vi "HandlingLargeDataset.vi"() -> ()   [LabVIEW 2019]
uses:
  <vilib>/addons/database/Connection.llb/DB Tools Open Connec (String).vi
  <vilib>/addons/database/Connection.llb/Conn Execute.vi
  <vilib>/addons/database/Recordset.llb/Rec Fetch Recordset Data (R).vi
  <vilib>/addons/database/_DB Variant To Data/Database Variant To Data.xnode
  <vilib>/addons/database/NI_Database_API.lvlib
panel:
  out "graph refreshed or not":bool
  out "x+y":timestamp
  out "element":timestamp
  out "max Date 1Hour":timestamp
  out "max Date 1 Month":timestamp
  out "max Date 1 week":timestamp
  out "max Date 30 minutes":timestamp
  out "max Date 1 Minute":timestamp
  out "max date 1Day":timestamp
  out "Horizontal":i32
  in  "To Date":timestamp
  in  "from Date":timestamp
  in  "Stop Button":bool
  in  "DateTime Array for One Month":timestamp[](array[timestamp])
  in  "Length Array for One Month":dbl[](array[numeric])
  out "concatenated string 8":string
  in  "DateTime Array for one week":timestamp[](array[timestamp])
  in  "Length Array for One week":dbl[](array[numeric])
  out "concatenated string 7":string
  in  "DateTime Array for 1 Day":timestamp[](array[timestamp])
  in  "Length Array for 1 Day":dbl[](array[numeric])
  out "concatenated string 6":string
  in  "DateTime Array for 1 Hour":timestamp[](array[timestamp])
  in  "Length Array for 1 Hour":dbl[](array[numeric])
  out "concatenated string 5":string
  out "concatenated string 2":string
  out "concatenated string":string
  out "Currently active btn":string
  in  "DateTime Array for 30 mins":timestamp[](array[timestamp])
  in  "Length Array for 30 mins":dbl[](array[numeric])
  out "record set data for 30 minutes":variant[][](array[variant])
  out "Month  3":string
  out "Day  3":string
  out "year  3":string
  out "Month  2":string
  out "Day  2":string
  out "year  2":string
  out "concatenated string 4":string
  out "NewVal":bool
  out "output cluster":T1
  out "DateTime Array  2":timestamp[](array[timestamp])
  in  "Length Array":dbl[](array[numeric])
  in  "DateTime Array":timestamp[](array[timestamp])
  out "size(s)":i32[](array[numeric])
  out "Month  2":string
  out "Day  2":string
  out "year  2":string
  out "Month":string
  out "Day":string
  out "year":string
  out "concatenated string 3":string
  in  "1Hour":bool
  in  "30Minute":bool
  in  "OneMinute":bool caption="One Minute"
  out "ZooM":T2(graph)
  in  "One Month":bool
  in  "One Week":bool
  in  "One Day":bool
  out "Tota records":variant[][](array[variant])
  out "Program start time":timestamp
  # "Welcome to History Section  for Data Analysis"
  # "One Week"
types:
  T1 = cluster{"DateTime Array ":timestamp[], "Length Array ":dbl[]}
  T2 = cluster{"DateTime from Db ":timestamp[], "start from Db ":dbl[]}
  T3 = typedef "LVPoint32TypeDef.ctl" = cluster{"Horizontal":i32, "Vertical":i32}
  T4 = typedef "NI_Database_API.lvlib/Conn ObjectReference.ctl" = refnum<k1>
  T5 = typedef "NI_Database_API.lvlib/Rec ObjectReference.ctl" = refnum<k1>
  T6 = cluster{"DateTime Array for 30 mins ":timestamp[], "Length Array for 30 mins ":dbl[]}
  T7 = cluster{"DateTime Array for one week ":timestamp[], "Length Array for One week":dbl[]}
  T8 = cluster{"DateTime Array for One Month ":timestamp[], "Length Array for One Month ":dbl[]}
  T9 = cluster{"DateTime Array for 1 Hour ":timestamp[], "Length Array for 1 Hour ":dbl[]}
  T10 = cluster{"DateTime Array for 1 Day ":timestamp[], "Length Array for 1 Day ":dbl[]}
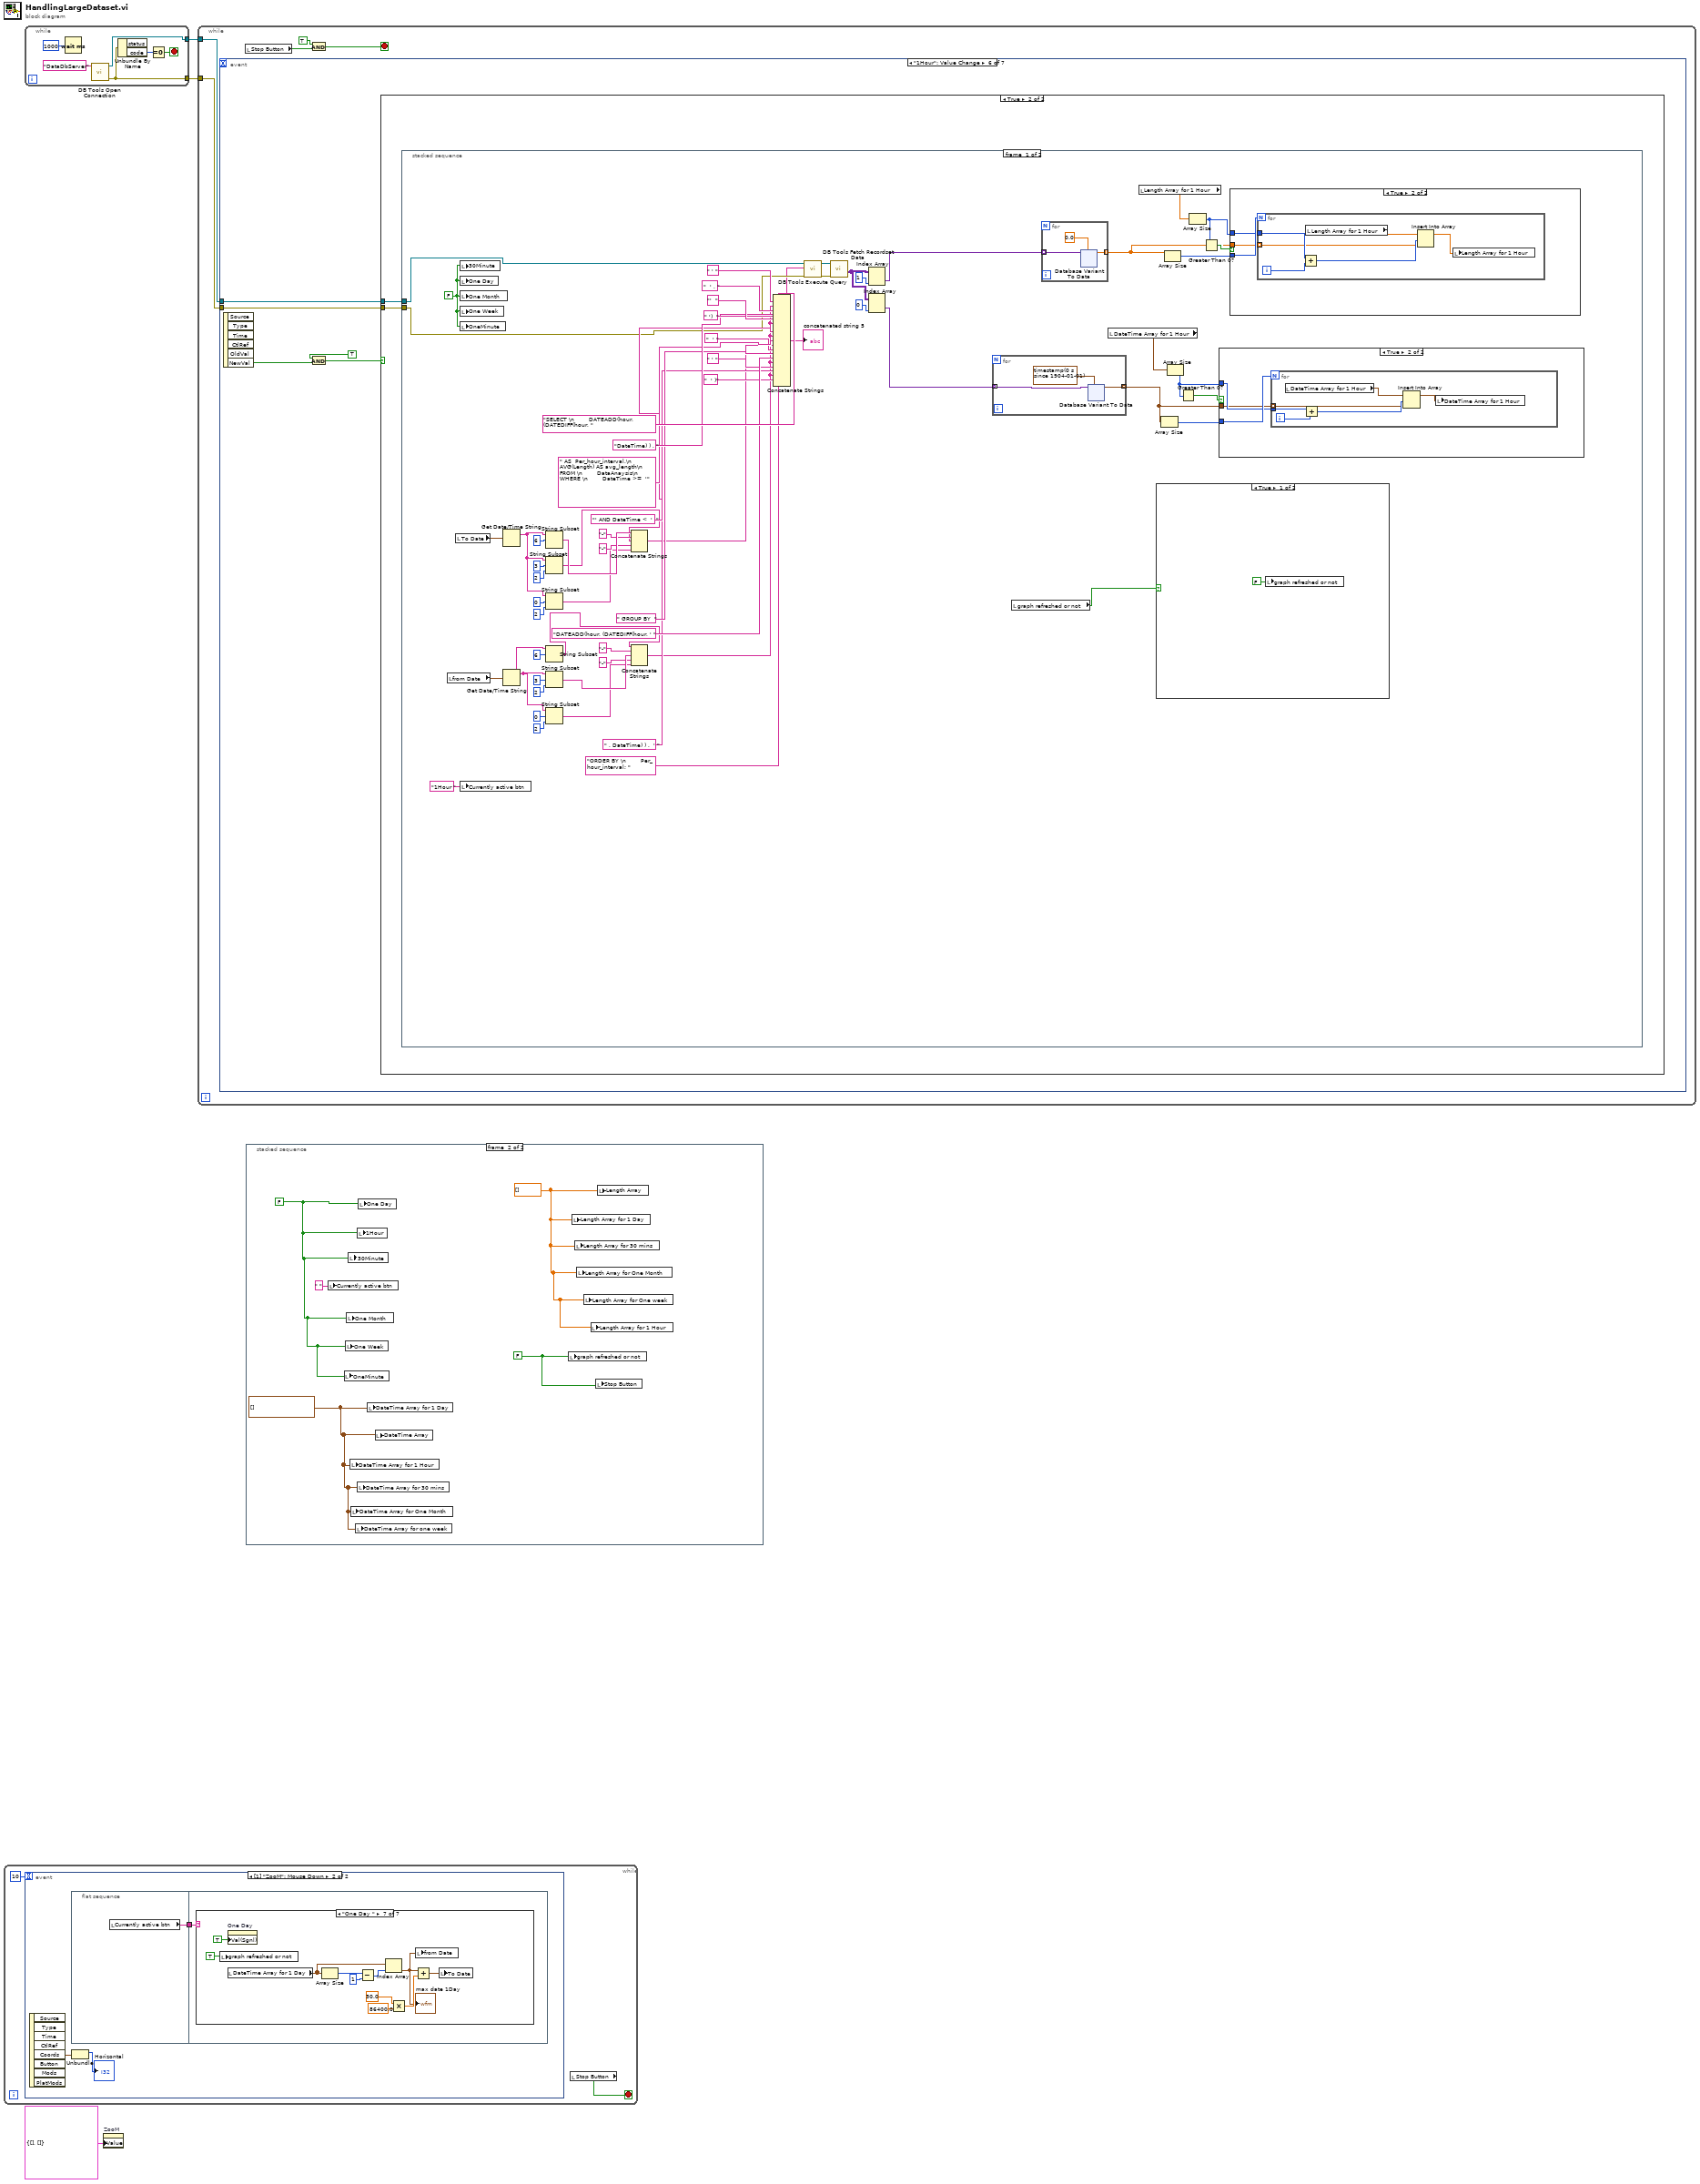
[diagram p0: block diagram]
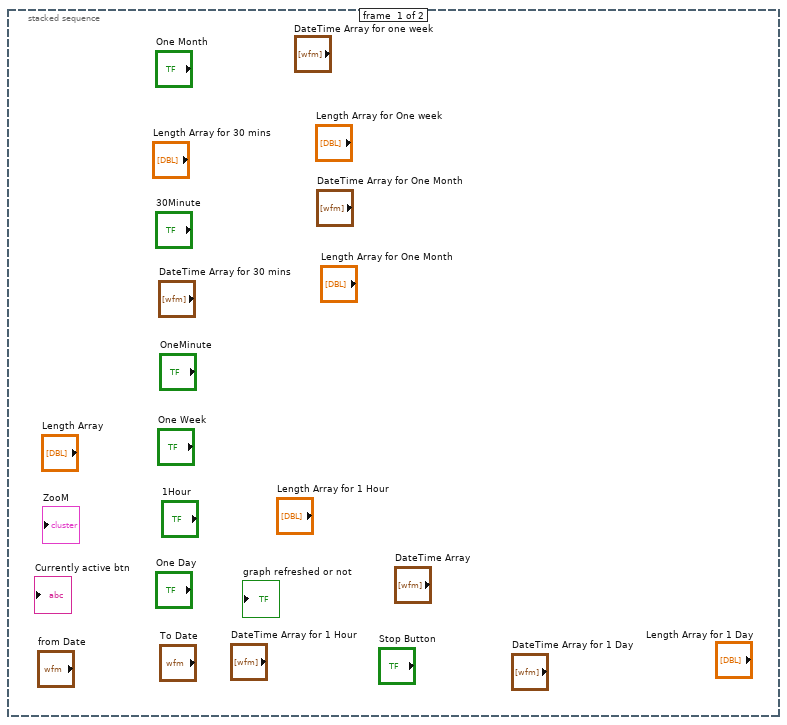
[diagram p2: hidden frame]
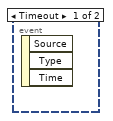
[diagram p3: hidden frame]
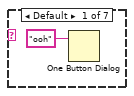
[diagram p4: hidden frame]
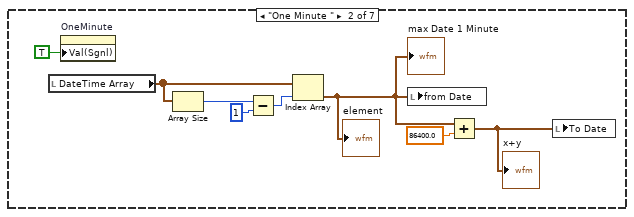
[diagram p5: hidden frame]
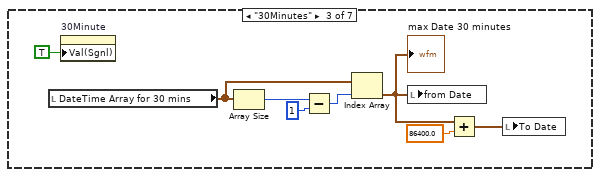
[diagram p6: hidden frame]
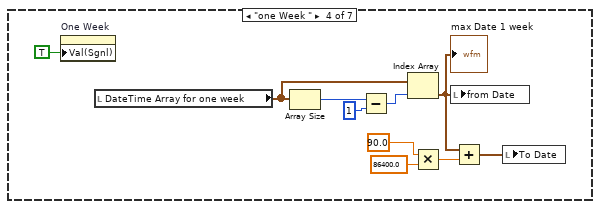
[diagram p7: hidden frame]
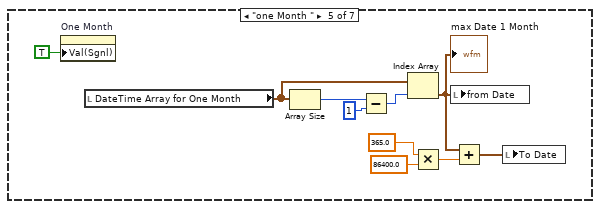
[diagram p8: hidden frame]
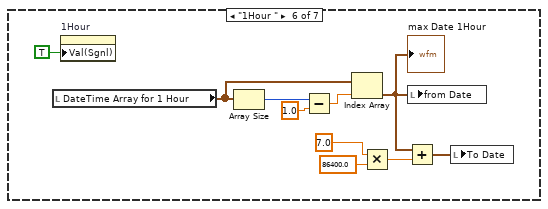
[diagram p9: hidden frame]
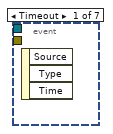
[diagram p10: hidden frame]
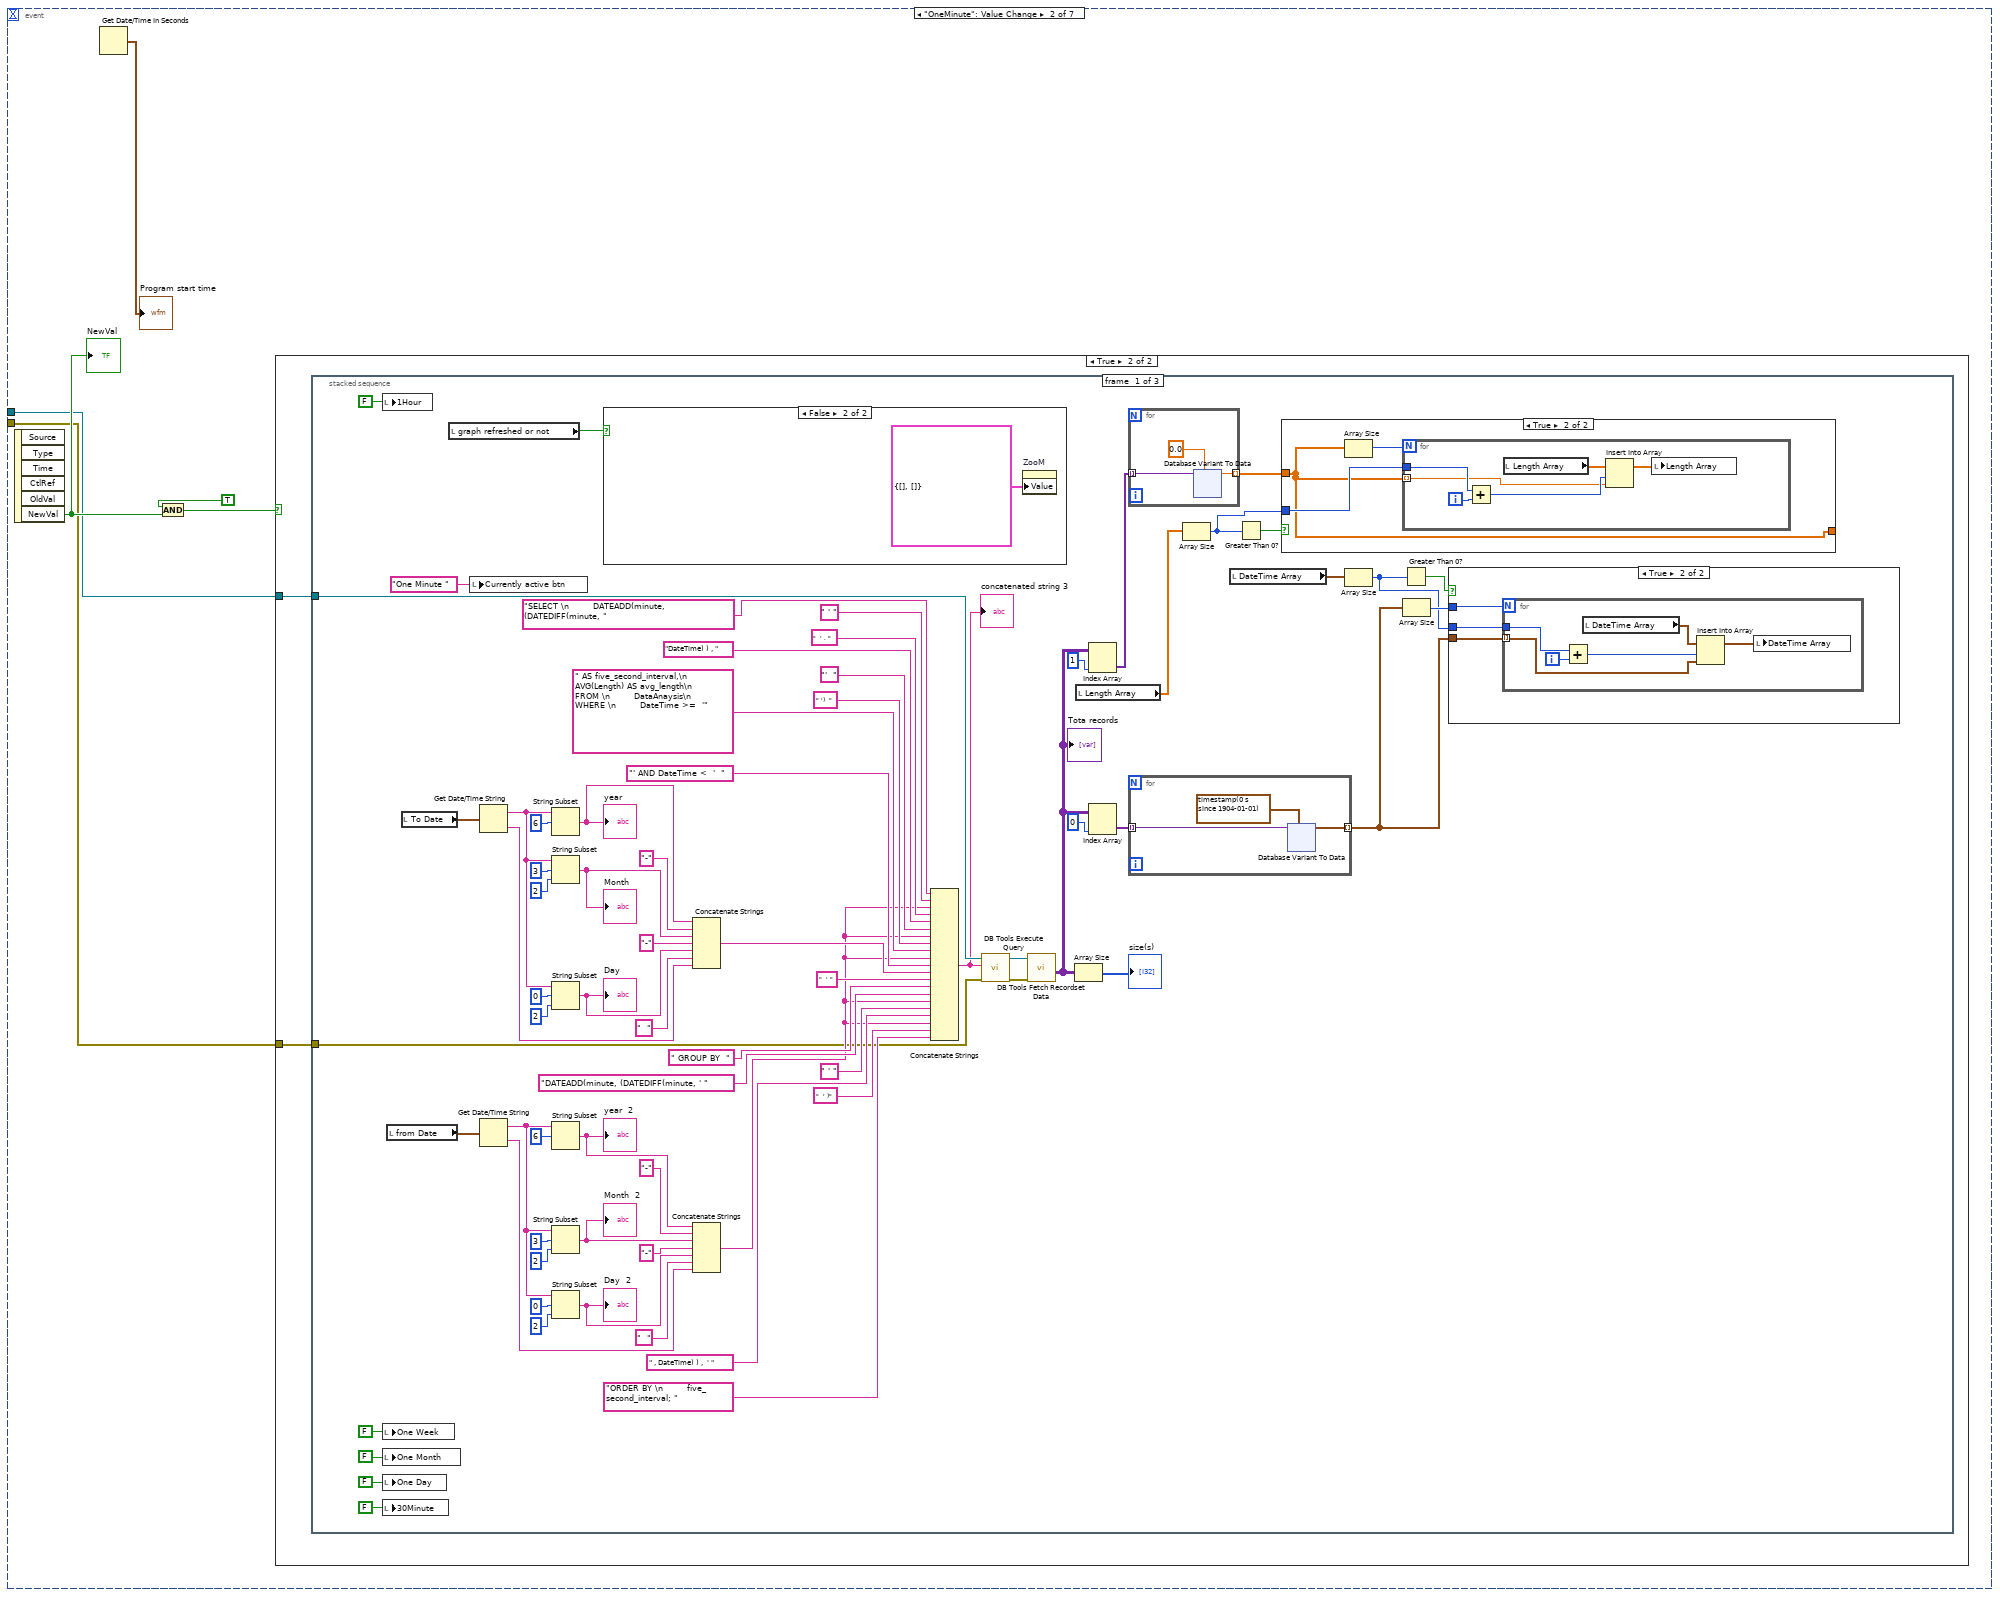
[diagram p11: hidden frame]
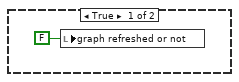
[diagram p13: hidden frame]
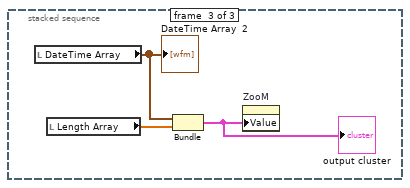
[diagram p17: hidden frame]
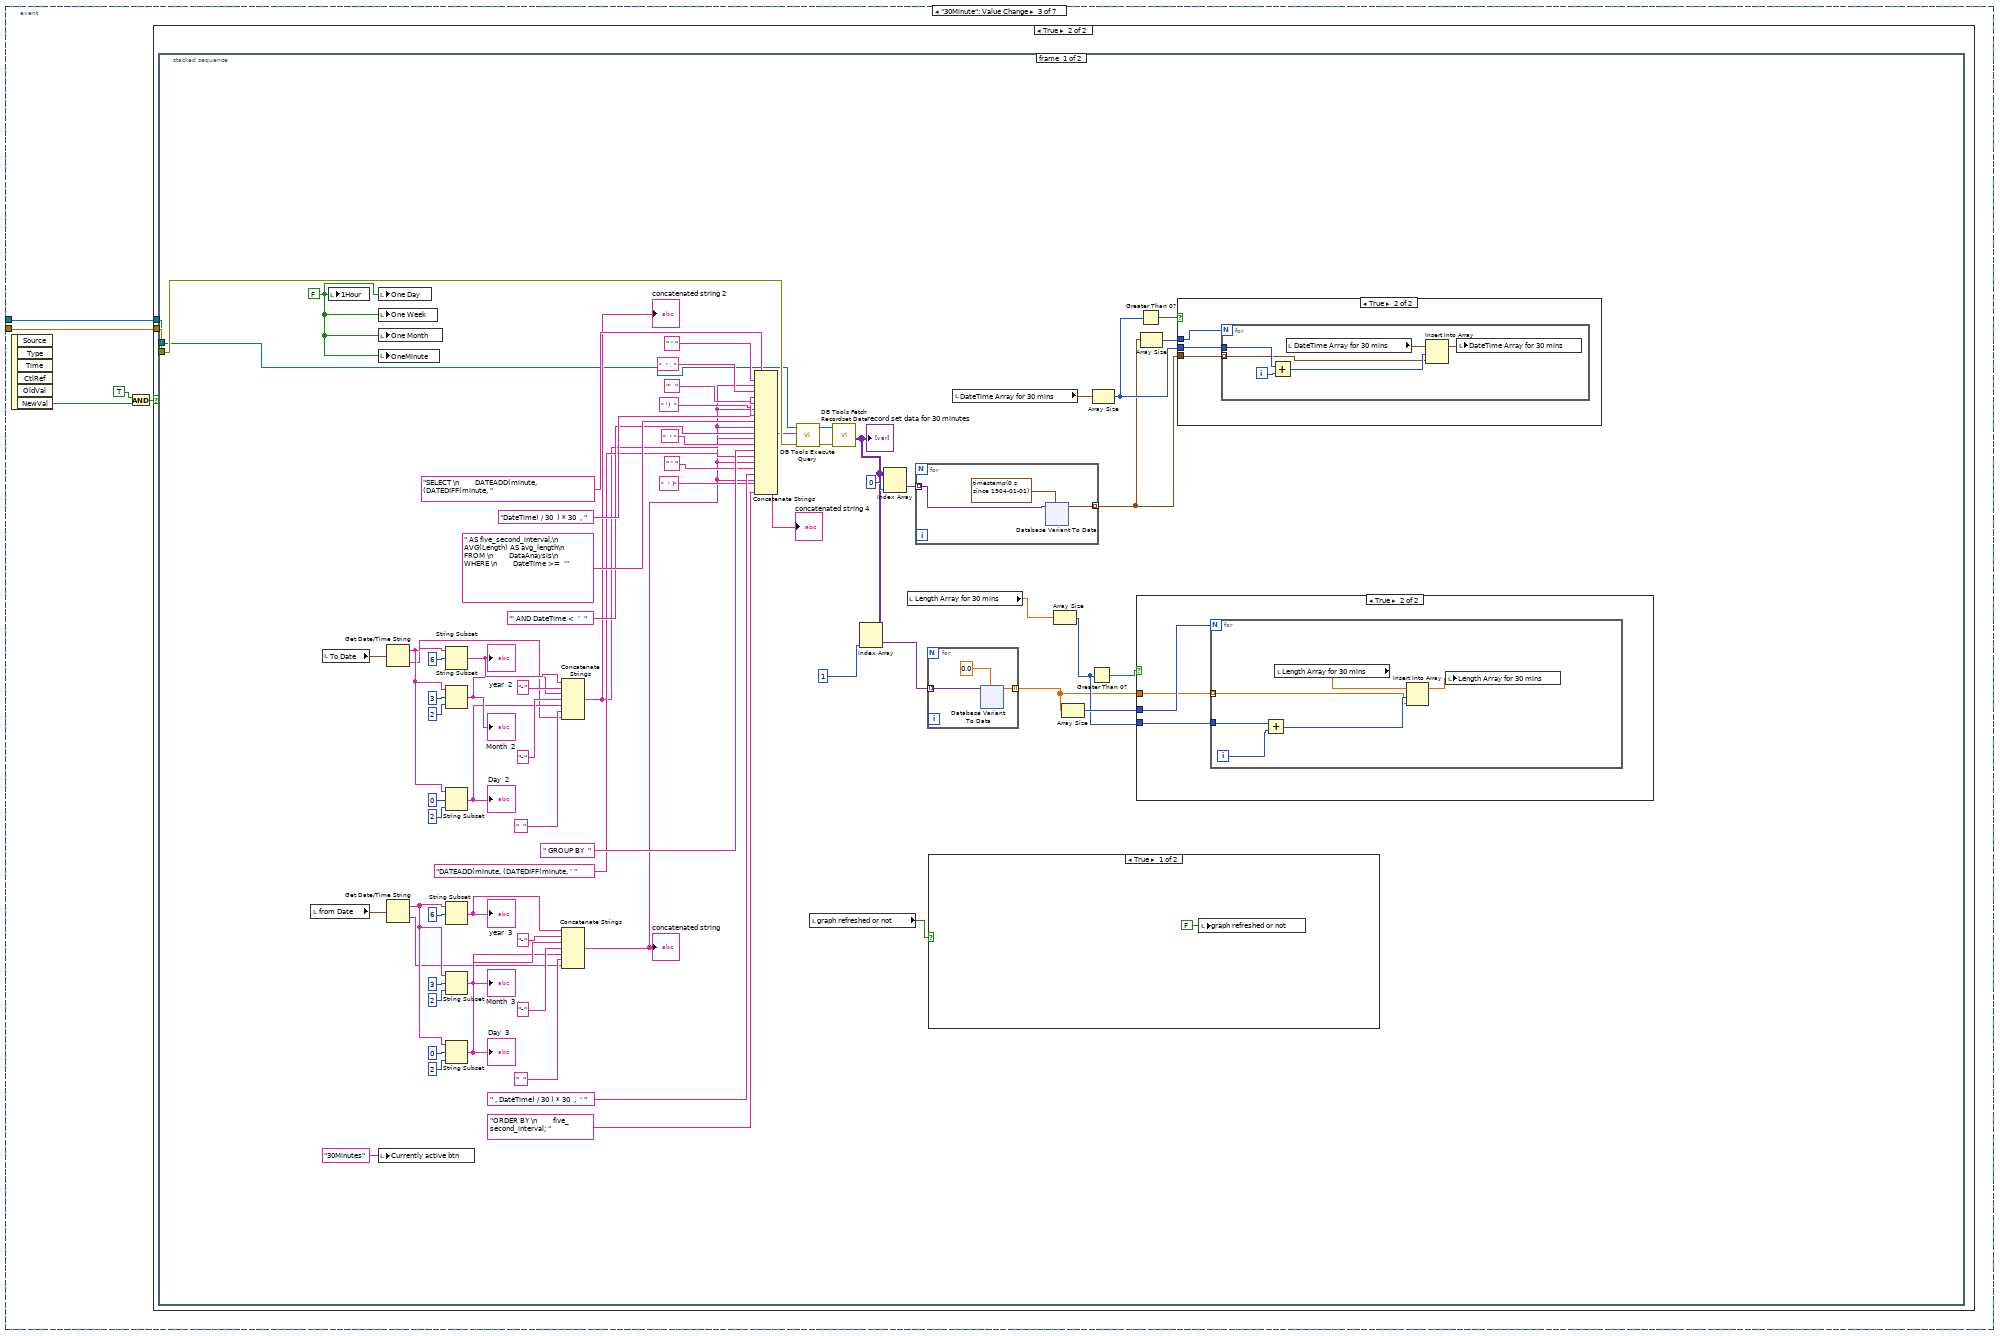
[diagram p18: hidden frame]
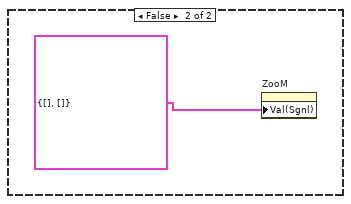
[diagram p20: hidden frame]
diagram:
  n1 = while {
    stop <- w4 stop-if-true
    n2 = event shown="[1] \"ZooM\": Mouse Down" {
      selector: _ -> [_ _]
      dyn-events: _ -> [_ _]
      timeout: 10 -> [_ _]
      event Timeout {
        n3 = event-data() -> ()  [unwired: 1 in, 3 out]
      }
      event "ZooM": Mouse Down {
        n4 = event-data() -> ("Coords"=w8:T3)  [unwired: 1 in, 7 out]
        n5 = flat-sequence {
          tunnel: [w9] -> w6
          tunnel: w6 -> [w10]
          frame #0 {
            n6 = local read "Currently active btn"() -> (w9:string)
          }
          frame #1 {
            n7 = case shown="\"One Day \"" w10 {
              frame Default {
                n8 = One Button Dialog(message="ooh") -> ()  [unwired: 1 in, 1 out]
              }
              frame "One Minute " {
                n9 = local read "DateTime Array"() -> (w19:timestamp[])
                n10 = property on="OneMinute" class="Bool (strict)"("Val(Sgnl)"=TRUE ("Value (Signaling)")) -> ()  [unwired: 2 in, 2 out]
                n11 = Array Size(array=w19) -> (size(s)=w17:i32)
                n12 = Subtract(x=w17, y=1) -> (x-y=w18:i32)
                n13 = Index Array(array=w19, index=w18) -> (element=w15:timestamp)
                "max Date 1 Minute" <- w15
                "element" <- w15
                n14 = local write "from Date"(w15) -> ()
                n15 = Add(x=w15, y=86400.0) -> (x+y=w13:timestamp)
                "x+y" <- w13
                n16 = local write "To Date"(w13) -> ()
              }
              frame "30Minutes" {
                n17 = local read "DateTime Array for 30 mins"() -> (w27:timestamp[])
                n18 = property on="30Minute" class="Bool (strict)"("Val(Sgnl)"=TRUE ("Value (Signaling)")) -> ()  [unwired: 2 in, 2 out]
                n19 = Array Size(array=w27) -> (size(s)=w26:i32)
                n20 = Subtract(x=w26, y=1) -> (x-y=w24:i32)
                n21 = Index Array(array=w27, index=w24) -> (element=w23:timestamp)
                "max Date 30 minutes" <- w23
                n22 = local write "from Date"(w23) -> ()
                n23 = Add(x=w23, y=86400.0) -> (x+y=w21:timestamp)
                n24 = local write "To Date"(w21) -> ()
              }
              frame "one Week " {
                n25 = property on="One Week" class="Bool (strict)"("Val(Sgnl)"=TRUE ("Value (Signaling)")) -> ()  [unwired: 2 in, 2 out]
                n26 = local read "DateTime Array for one week"() -> (w35:timestamp[])
                n27 = Array Size(array=w35) -> (size(s)=w37:i32)
                n28 = Subtract(x=w37, y=1) -> (x-y=w34:i32)
                n29 = Index Array(array=w35, index=w34) -> (element=w33:timestamp)
                "max Date 1 week" <- w33
                n30 = Multiply(x=90.0, y=86400.0) -> (x*y=w30:dbl)
                n31 = local write "from Date"(w33) -> ()
                n32 = Add(x=w33, y=w30) -> (x+y=w29:timestamp)
                n33 = local write "To Date"(w29) -> ()
              }
              frame "one Month " {
                n34 = property on="One Month" class="Bool (strict)"("Val(Sgnl)"=TRUE ("Value (Signaling)")) -> ()  [unwired: 2 in, 2 out]
                n35 = local read "DateTime Array for One Month"() -> (w44:timestamp[])
                n36 = Array Size(array=w44) -> (size(s)=w47:i32)
                n37 = Subtract(x=w47, y=1) -> (x-y=w45:i32)
                n38 = Index Array(array=w44, index=w45) -> (element=w43:timestamp)
                "max Date 1 Month" <- w43
                n39 = Multiply(x=365.0, y=86400.0) -> (x*y=w40:dbl)
                n40 = local write "from Date"(w43) -> ()
                n41 = Add(x=w43, y=w40) -> (x+y=w39:timestamp)
                n42 = local write "To Date"(w39) -> ()
              }
              frame "1Hour " {
                n43 = local read "DateTime Array for 1 Hour"() -> (w54:timestamp[])
                n44 = property on="1Hour" class="Bool (strict)"("Val(Sgnl)"=TRUE ("Value (Signaling)")) -> ()  [unwired: 2 in, 2 out]
                n45 = Array Size(array=w54) -> (size(s)=w55:i32)
                n46 = Subtract(x=w55, y=1.0) -> (x-y=w57:dbl)
                n47 = Index Array(array=w54, index=w57) -> (element=w50:timestamp)
                "max Date 1Hour" <- w50
                n48 = Multiply(x=7.0, y=86400.0) -> (x*y=w51:dbl)
                n49 = Add(x=w50, y=w51) -> (x+y=w49:timestamp)
                n50 = local write "from Date"(w50) -> ()
                n51 = local write "To Date"(w49) -> ()
              }
              frame "One Day " {
                n52 = local write "graph refreshed or not"(TRUE ("graph refreshed or not")) -> ()
                n53 = property on="One Day" class="Bool (strict)"("Val(Sgnl)"=TRUE ("Value (Signaling)")) -> ()  [unwired: 2 in, 2 out]
                n54 = local read "DateTime Array for 1 Day"() -> (w68:timestamp[])
                n55 = Array Size(array=w68) -> (size(s)=w66:i32)
                n56 = Subtract(x=w66, y=1) -> (x-y=w67:i32)
                n57 = Index Array(array=w68, index=w67) -> (element=w61:timestamp)
                "max date 1Day" <- w61
                n58 = Multiply(x=30.0, y=86400.0) -> (x*y=w62:dbl)
                n59 = Add(x=w61, y=w62) -> (x+y=w60:timestamp)
                n60 = local write "from Date"(w61) -> ()
                n61 = local write "To Date"(w60) -> ()
              }
            }
          }
        }
        n62 = Unbundle(w8) -> ("Horizontal"=→"Horizontal":i32)  [unwired: 1 out]
      }
    }
    n63 = local read "Stop Button"() -> (w4:bool)
  }
  n64 = while {
    tunnel: [w70] -> w1
    tunnel: [w72] -> w2
    stop <- w69 stop-if-true
    n65 = Wait (ms)(milliseconds to wait=u32 1000) -> ()  [unwired: 1 out]
    n66 = call-poly <vilib>:"DB Tools Open Connection.vi"("connection information"="DataDbServer") -> ("error out"=w72:errorcluster, "connection reference"=w70:T4)  [unwired: 7 in]
    n67 = Unbundle By Name(w72) -> ("code"=w73:i32)  [unwired: 1 out]
    n68 = Equal To 0?(x=w73) -> (x = 0?=w69:bool)
  }
  n69 = property on="ZooM" class="XYGraph (strict)"("Value"=cluster{timestamp[], dbl[]} {[], []}) -> ()  [unwired: 2 in, 2 out]
  n70 = while {
    tunnel: w2 -> [w79]
    tunnel: w1 -> [w78]
    stop <- w75 stop-if-true
    n71 = event shown="[5] \"1Hour\": Value Change" {
      selector: _ -> [_ _ _ _ _ _ _]
      dyn-events: _ -> [_ _ _ _ _ _ _]
      timeout: _ -> [_ _ _ _ _ _ _]
      tunnel: w79 -> [_ w80 w267 w450 w627 w805 w984]
      tunnel: w78 -> [_ w81 w266 w449 w626 w804 w983]
      event Timeout {
        n72 = event-data() -> ()  [unwired: 1 in, 3 out]
      }
      event "OneMinute": Value Change {
        n73 = event-data() -> ("NewVal"=w83:bool)  [unwired: 1 in, 5 out]
        "NewVal" <- w83
        n74 = Get Date/Time In Seconds() -> (seconds since 1Jan1904=→"Program start time":timestamp)
        n75 = And(x=TRUE, y=w83) -> (x .and. y?=w82:bool)
        n76 = case shown="True" w82 {
          tunnel: w81 -> [_ w87]
          tunnel: w80 -> [_ w86]
          frame False {
          }
          frame True {
            n77 = stacked-sequence {
              tunnel: w87 -> [w115 _ _]
              tunnel: w86 -> [w116 _ _]
              frame #0 {
                n78 = local write "1Hour"(FALSE ("1Hour")) -> ()
                n79 = local write "One Week"(FALSE ("One Week")) -> ()
                n80 = local write "One Month"(FALSE ("One Month")) -> ()
                n81 = local write "One Day"(FALSE ("One Day")) -> ()
                n82 = local write "30Minute"(FALSE ("30Minute")) -> ()
                n83 = local read "from Date"() -> (w144:timestamp)
                n84 = local read "To Date"() -> (w143:timestamp)
                n85 = local read "graph refreshed or not"() -> (w88:bool)
                n86 = local write "Currently active btn"("One Minute ") -> ()
                n87 = Get Date/Time String(seconds (now)=w143) -> (date string=w137:string, time string=w98:string)  [unwired: 2 in]
                n88 = Get Date/Time String(seconds (now)=w144) -> (date string=w120:string, time string=w100:string)  [unwired: 2 in]
                n89 = String Subset(string=w137, offset (0)=6) -> (substring=w136:string)  [unwired: 1 in]
                "year" <- w136
                n90 = String Subset(string=w137, offset (0)=3, length (rest)=2 ("length (rest)")) -> (substring=w134:string)
                "Month" <- w134
                n91 = String Subset(string=w137, offset (0)=0, length (rest)=2 ("length (rest)")) -> (substring=w132:string)
                "Day" <- w132
                n92 = String Subset(string=w120, offset (0)=6) -> (substring=w125:string)  [unwired: 1 in]
                "year  2" <- w125
                n93 = String Subset(string=w120, offset (0)=3, length (rest)=2 ("length (rest)")) -> (substring=w123:string)
                "Month  2" <- w123
                n94 = String Subset(string=w120, offset (0)=0, length (rest)=2 ("length (rest)")) -> (substring=w121:string)
                "Day  2" <- w121
                n95 = case shown="False" w88 {
                  frame True {
                    n96 = local write "graph refreshed or not"(FALSE ("graph refreshed or not")) -> ()
                  }
                  frame False {
                    n97 = property on="ZooM" class="XYGraph (strict)"("Value"=cluster{timestamp[], dbl[]} {[], []}) -> ()  [unwired: 2 in, 2 out]
                  }
                }
                n98 = Concatenate Strings(w136, "-" ("string"), w134, "-" ("string"), w132, "  " ("string"), w98) -> (w131:string)
                n99 = Concatenate Strings(w125, "-" ("string"), w123, "-" ("string"), w121, "  " ("string"), w100) -> (w119:string)
                n100 = Concatenate Strings("SELECT \n        DATEADD(minute, (DATEDIFF(minute, " ("string"), " ' " ("string"), w119, "  ' , " ("string"), "DateTime) ) , " ("string"), "'  " ("string"), w119, " ')  " ("string"), " AS five_second_interval,\n        AVG(Length) AS avg_length\n    FROM \n        DataAnaysis\n    WHERE \n        DateTime >=  '" ("string"), w119, "' AND DateTime <  '  " ("string"), w131, "  ' " ("string"), " GROUP BY  " ("string"), "DATEADD(minute, (DATEDIFF(minute, ' " ("string"), w119, " ' " ("string"), " , DateTime) ) ,  ' " ("string"), w119, "  ' )" ("string"), "ORDER BY \n        five_second_interval; " ("string")) -> (w114:string)
                "concatenated string 3" <- w114
                n101 = call-poly <vilib>:"DB Tools Execute Query.vi"("error in (no error)"=w116, "SQL query"=w114, "connection reference"=w115) -> ("error out"=w117:errorcluster, "recordset reference"=w118:T5)  [unwired: 5 in]
                n102 = call-poly <vilib>:"DB Tools Fetch Recordset Data.vi"("error in (no error)"=w117, "recordset reference"=w118) -> ("recordset data"=w110:variant[][])  [unwired: 3 in, 2 out]
                "Tota records" <- w110
                n103 = Array Size(array=w110) -> (size(s)=→"size(s)":i32[])
                n104 = local read "Length Array"() -> (w97:dbl[])
                n105 = Index Array(array=w110, index (col)=1 ("disabled index (col)")) -> (element=w108:variant[])  [unwired: 1 in]
                n106 = Index Array(array=w110, index (col)=0 ("disabled index (col)")) -> (element=w111:variant[])  [unwired: 1 in]
                n107 = for {
                  tunnel: w108 -> [w182] mode=indexing
                  tunnel: [w180] -> w95 mode=indexing
                  n108 = xnode "Database Variant To Data"("database variant"=w182, "type"=0.0) -> ("data"=w180:dbl)  [unwired: 1 in, 1 out]
                }
                n109 = for {
                  tunnel: w111 -> [w217] mode=indexing
                  tunnel: [w215] -> w89 mode=indexing
                  n110 = xnode "Database Variant To Data"("database variant"=w217, "type"=timestamp(0 s since 1904-01-01)) -> ("data"=w215:timestamp)  [unwired: 1 in, 1 out]
                }
                n111 = Array Size(array=w97) -> (size(s)=w94:i32)
                n112 = local read "DateTime Array"() -> (w93:timestamp[])
                n113 = Greater Than 0?(x=w94) -> (x > 0?=w96:bool)
                n114 = case shown="True" w96 {
                  tunnel: [_ w171] -> _
                  tunnel: w95 -> [_ w171]
                  tunnel: w94 -> [_ w172]
                  frame False {
                  }
                  frame True {
                    n115 = Array Size(array=w171) -> (size(s)=w173:i32)
                    n116 = for {
                      N: w173 -> [_]
                      tunnel: w172 -> [w177]
                      tunnel: w171 -> [w175] mode=indexing
                      i -> [w178]
                      n117 = Add(x=w177, y=w178) -> (x+y=w176:i32)
                      n118 = local read "Length Array"() -> (w179:dbl[])
                      n119 = Insert Into Array(array=w179, index=w176, new element=w175) -> (w174:dbl[])
                      n120 = local write "Length Array"(w174) -> ()
                    }
                  }
                }
                n121 = Array Size(array=w93) -> (size(s)=w90:i32)
                n122 = Greater Than 0?(x=w90) -> (x > 0?=w92:bool)
                n123 = Array Size(array=w89) -> (size(s)=w91:i32)
                n124 = case shown="True" w92 {
                  tunnel: w91 -> [_ w164]
                  tunnel: w90 -> [_ w163]
                  tunnel: w89 -> [_ w162]
                  frame False {
                  }
                  frame True {
                    n125 = for {
                      N: w164 -> [_]
                      tunnel: w163 -> [w168]
                      tunnel: w162 -> [w166] mode=indexing
                      i -> [w169]
                      n126 = Add(x=w168, y=w169) -> (x+y=w167:i32)
                      n127 = local read "DateTime Array"() -> (w170:timestamp[])
                      n128 = Insert Into Array(array=w170, index=w167, new element=w166) -> (w165:timestamp[])
                      n129 = local write "DateTime Array"(w165) -> ()
                    }
                  }
                }
              }
              frame #1 {
              }
              frame #2 {
                n130 = local read "DateTime Array"() -> (w265:timestamp[])
                "DateTime Array  2" <- w265
                n131 = local read "Length Array"() -> (w264:dbl[])
                n132 = Bundle("DateTime Array"=w265, "Length Array"=w264) -> (w263:T1)  [unwired: 1 in]
                "output cluster" <- w263
                n133 = property on="ZooM" class="XYGraph (strict)"("Value"=w263) -> ()  [unwired: 2 in, 2 out]
              }
            }
          }
        }
      }
      event "30Minute": Value Change {
        n134 = event-data() -> ("NewVal"=w270:bool)  [unwired: 1 in, 5 out]
        n135 = And(x=TRUE, y=w270) -> (x .and. y?=w268:bool)
        n136 = case shown="True" w268 {
          tunnel: w267 -> [_ w272]
          tunnel: w266 -> [_ w271]
          frame False {
          }
          frame True {
            n137 = stacked-sequence {
              tunnel: w272 -> [w300 _]
              tunnel: w271 -> [w299 _]
              frame #0 {
                w288 = FALSE ("1Hour")
                n138 = local read "from Date"() -> (w326:timestamp)
                n139 = local read "To Date"() -> (w325:timestamp)
                n140 = local write "1Hour"(w288) -> ()
                n141 = local write "One Day"(w288) -> ()
                n142 = local write "One Week"(w288) -> ()
                n143 = local write "One Month"(w288) -> ()
                n144 = local write "OneMinute"(w288) -> ()
                n145 = local write "Currently active btn"("30Minutes") -> ()
                n146 = Get Date/Time String(seconds (now)=w325) -> (date string=w319:string, time string=w284:string)  [unwired: 2 in]
                n147 = Get Date/Time String(seconds (now)=w326) -> (date string=w302:string, time string=w286:string)  [unwired: 2 in]
                n148 = String Subset(string=w319, offset (0)=6) -> (substring=w318:string)  [unwired: 1 in]
                "year  2" <- w318
                n149 = String Subset(string=w319, offset (0)=3, length (rest)=2 ("length (rest)")) -> (substring=w316:string)
                "Month  2" <- w316
                n150 = String Subset(string=w319, offset (0)=0, length (rest)=2 ("length (rest)")) -> (substring=w314:string)
                "Day  2" <- w314
                n151 = String Subset(string=w302, offset (0)=6) -> (substring=w301:string)  [unwired: 1 in]
                "year  3" <- w301
                n152 = String Subset(string=w302, offset (0)=3, length (rest)=2 ("length (rest)")) -> (substring=w307:string)
                "Month  3" <- w307
                n153 = String Subset(string=w302, offset (0)=0, length (rest)=2 ("length (rest)")) -> (substring=w305:string)
                "Day  3" <- w305
                n154 = Concatenate Strings(w318, "-" ("string"), w316, "-" ("string"), w314, "  " ("string"), w284) -> (w313:string)
                "concatenated string 2" <- w313
                n155 = Concatenate Strings(w301, "-" ("string"), w307, "-" ("string"), w305, "  " ("string"), w286) -> (w304:string)
                "concatenated string" <- w304
                n156 = Concatenate Strings("SELECT \n        DATEADD(minute, (DATEDIFF(minute, " ("string"), " ' " ("string"), w304, "  ' , " ("string"), "DateTime) / 30  ) * 30  , " ("string"), "'  " ("string"), w304, " ')  " ("string"), " AS five_second_interval,\n        AVG(Length) AS avg_length\n    FROM \n        DataAnaysis\n    WHERE \n        DateTime >=  '" ("string"), w304, "' AND DateTime <  '  " ("string"), w313, "  ' " ("string"), " GROUP BY  " ("string"), "DATEADD(minute, (DATEDIFF(minute, ' " ("string"), w304, " ' " ("string"), " , DateTime) / 30 ) * 30  ,  ' " ("string"), w304, "  ' )" ("string"), "ORDER BY \n        five_second_interval; " ("string")) -> (w298:string)
                "concatenated string 4" <- w298
                n157 = call-poly <vilib>:"DB Tools Execute Query.vi"("error in (no error)"=w300, "SQL query"=w298, "connection reference"=w299) -> ("error out"=w297:errorcluster, "recordset reference"=w296:T5)  [unwired: 5 in]
                n158 = local read "graph refreshed or not"() -> (w273:bool)
                n159 = call-poly <vilib>:"DB Tools Fetch Recordset Data.vi"("error in (no error)"=w297, "recordset reference"=w296) -> ("recordset data"=w291:variant[][])  [unwired: 3 in, 2 out]
                "record set data for 30 minutes" <- w291
                n160 = Index Array(array=w291, index (col)=1 ("disabled index (col)")) -> (element=w292:variant[])  [unwired: 1 in]
                n161 = Index Array(array=w291, index (col)=0 ("disabled index (col)")) -> (element=w294:variant[])  [unwired: 1 in]
                n162 = local read "Length Array for 30 mins"() -> (w277:dbl[])
                n163 = for {
                  tunnel: w294 -> [w400] mode=indexing
                  tunnel: [w398] -> w279 mode=indexing
                  n164 = xnode "Database Variant To Data"("database variant"=w400, "type"=timestamp(0 s since 1904-01-01)) -> ("data"=w398:timestamp)  [unwired: 1 in, 1 out]
                }
                n165 = for {
                  tunnel: w292 -> [w365] mode=indexing
                  tunnel: [w363] -> w274 mode=indexing
                  n166 = xnode "Database Variant To Data"("database variant"=w365, "type"=0.0) -> ("data"=w363:dbl)  [unwired: 1 in, 1 out]
                }
                n167 = case shown="True" w273 {
                  frame True {
                    n168 = local write "graph refreshed or not"(FALSE ("graph refreshed or not")) -> ()
                  }
                  frame False {
                    n169 = property on="ZooM" class="XYGraph (strict)"("Val(Sgnl)"=cluster{timestamp[], dbl[]} {[], []}) -> ()  [unwired: 2 in, 2 out]
                  }
                }
                n170 = local read "DateTime Array for 30 mins"() -> (w283:timestamp[])
                n171 = Array Size(array=w277) -> (size(s)=w275:i32)
                n172 = Array Size(array=w274) -> (size(s)=w276:i32)
                n173 = Greater Than 0?(x=w275) -> (x > 0?=w278:bool)
                n174 = Array Size(array=w283) -> (size(s)=w280:i32)
                n175 = case shown="True" w278 {
                  tunnel: w276 -> [_ w346]
                  tunnel: w275 -> [_ w345]
                  tunnel: w274 -> [w343 w344]
                  frame False {
                    n176 = local write "Length Array for 30 mins"(w343) -> ()
                  }
                  frame True {
                    n177 = for {
                      N: w346 -> [_]
                      tunnel: w345 -> [w350]
                      tunnel: w344 -> [w348] mode=indexing
                      i -> [w351]
                      n178 = Add(x=w350, y=w351) -> (x+y=w349:i32)
                      n179 = local read "Length Array for 30 mins"() -> (w352:dbl[])
                      n180 = Insert Into Array(array=w352, index=w349, new element=w348) -> (w347:dbl[])
                      n181 = local write "Length Array for 30 mins"(w347) -> ()
                    }
                  }
                }
                n182 = Greater Than 0?(x=w280) -> (x > 0?=w282:bool)
                n183 = Array Size(array=w279) -> (size(s)=w281:i32)
                n184 = case shown="True" w282 {
                  tunnel: w281 -> [_ w356]
                  tunnel: w280 -> [_ w355]
                  tunnel: w279 -> [w353 w354]
                  frame False {
                    n185 = local write "DateTime Array for 30 mins"(w353) -> ()
                  }
                  frame True {
                    n186 = for {
                      N: w356 -> [_]
                      tunnel: w355 -> [w360]
                      tunnel: w354 -> [w358] mode=indexing
                      i -> [w361]
                      n187 = Add(x=w360, y=w361) -> (x+y=w359:i32)
                      n188 = local read "DateTime Array for 30 mins"() -> (w362:timestamp[])
                      n189 = Insert Into Array(array=w362, index=w359, new element=w358) -> (w357:timestamp[])
                      n190 = local write "DateTime Array for 30 mins"(w357) -> ()
                    }
                  }
                }
              }
              frame #1 {
                n191 = local read "DateTime Array for 30 mins"() -> (w447:timestamp[])
                n192 = local read "Length Array for 30 mins"() -> (w448:dbl[])
                n193 = Bundle("DateTime Array for 30 mins"=w447, "Length Array for 30 mins"=w448) -> (w446:T6)  [unwired: 1 in]
                n194 = property on="ZooM" class="XYGraph (strict)"("Value"=w446) -> ()  [unwired: 2 in, 2 out]
              }
            }
          }
        }
      }
      event "One Week": Value Change {
        n195 = event-data() -> ("NewVal"=w453:bool)  [unwired: 1 in, 5 out]
        n196 = And(x=TRUE, y=w453) -> (x .and. y?=w451:bool)
        n197 = case shown="True" w451 {
          tunnel: w450 -> [_ w455]
          tunnel: w449 -> [_ w454]
          frame False {
          }
          frame True {
            n198 = stacked-sequence {
              tunnel: w455 -> [w476 _]
              tunnel: w454 -> [w475 _]
              frame #0 {
                w466 = FALSE ("1Hour")
                n199 = local read "from Date"() -> (w482:timestamp)
                n200 = local read "To Date"() -> (w481:timestamp)
                n201 = local write "1Hour"(w466) -> ()
                n202 = local write "One Day"(w466) -> ()
                n203 = local write "OneMinute"(w466) -> ()
                n204 = local write "One Month"(w466) -> ()
                n205 = local write "30Minute"(w466) -> ()
                n206 = local write "Currently active btn"("one Week ") -> ()
                n207 = Get Date/Time String(seconds (now)=w481) -> (date string=w498:string)  [unwired: 2 in, 1 out]
                n208 = Get Date/Time String(seconds (now)=w482) -> (date string=w479:string)  [unwired: 2 in, 1 out]
                n209 = String Subset(string=w498, offset (0)=6) -> (substring=w497:string)  [unwired: 1 in]
                n210 = String Subset(string=w498, offset (0)=3, length (rest)=2 ("length (rest)")) -> (substring=w495:string)
                n211 = String Subset(string=w498, offset (0)=0, length (rest)=2 ("length (rest)")) -> (substring=w493:string)
                n212 = String Subset(string=w479, offset (0)=6) -> (substring=w477:string)  [unwired: 1 in]
                n213 = String Subset(string=w479, offset (0)=3, length (rest)=2 ("length (rest)")) -> (substring=w486:string)
                n214 = String Subset(string=w479, offset (0)=0, length (rest)=2 ("length (rest)")) -> (substring=w484:string)
                n215 = Concatenate Strings(w497, "-" ("string"), w495, "-" ("string"), w493) -> (w492:string)
                n216 = Concatenate Strings(w477, "-" ("string"), w486, "-" ("string"), w484) -> (w483:string)
                n217 = Concatenate Strings("SELECT \n        DATEADD(week, (DATEDIFF(week , " ("string"), " ' " ("string"), w483, "  ' , " ("string"), "DateTime) ) , " ("string"), "'  " ("string"), w483, " ')  " ("string"), " AS  Per_week_interval,\n        AVG(Length) AS avg_length\n    FROM \n        DataAnaysis\n    WHERE \n        DateTime >=  '" ("string"), w483, "' AND DateTime <  '  " ("string"), w492, "  ' " ("string"), " GROUP BY  " ("string"), "DATEADD(week, (DATEDIFF(week, ' " ("string"), w483, " ' " ("string"), " , DateTime) ) ,  ' " ("string"), w483, "  ' )" ("string"), "ORDER BY \n        Per_week_interval; " ("string")) -> (w472:string)
                "concatenated string 7" <- w472
                n218 = local read "DateTime Array for one week"() -> (w465:timestamp[])
                n219 = call-poly <vilib>:"DB Tools Execute Query.vi"("error in (no error)"=w476, "SQL query"=w472, "connection reference"=w475) -> ("error out"=w474:errorcluster, "recordset reference"=w473:T5)  [unwired: 5 in]
                n220 = call-poly <vilib>:"DB Tools Fetch Recordset Data.vi"("error in (no error)"=w474, "recordset reference"=w473) -> ("recordset data"=w467:variant[][])  [unwired: 3 in, 2 out]
                n221 = Array Size(array=w465) -> (size(s)=w462:i32)
                n222 = Greater Than 0?(x=w462) -> (x > 0?=w464:bool)
                n223 = Index Array(array=w467, index (col)=1 ("disabled index (col)")) -> (element=w468:variant[])  [unwired: 1 in]
                n224 = Index Array(array=w467, index (col)=0 ("disabled index (col)")) -> (element=w470:variant[])  [unwired: 1 in]
                n225 = for {
                  tunnel: w470 -> [w577] mode=indexing
                  tunnel: [w575] -> w461 mode=indexing
                  n226 = xnode "Database Variant To Data"("database variant"=w577, "type"=timestamp(0 s since 1904-01-01)) -> ("data"=w575:timestamp)  [unwired: 1 in, 1 out]
                }
                n227 = Array Size(array=w461) -> (size(s)=w463:i32)
                n228 = case shown="False" w464 {
                  tunnel: w463 -> [_ w533]
                  tunnel: w462 -> [_ w532]
                  tunnel: w461 -> [w530 w531]
                  frame False {
                    n229 = local write "DateTime Array for one week"(w530) -> ()
                  }
                  frame True {
                    n230 = for {
                      N: w533 -> [_]
                      tunnel: w532 -> [w537]
                      tunnel: w531 -> [w535] mode=indexing
                      i -> [w538]
                      n231 = local read "DateTime Array for one week"() -> (w539:timestamp[])
                      n232 = Add(x=w537, y=w538) -> (x+y=w536:i32)
                      n233 = Insert Into Array(array=w539, index=w536, new element=w535) -> (w534:timestamp[])
                      n234 = local write "DateTime Array for one week"(w534) -> ()
                    }
                  }
                }
                n235 = for {
                  tunnel: w468 -> [w542] mode=indexing
                  tunnel: [w540] -> w458 mode=indexing
                  n236 = xnode "Database Variant To Data"("database variant"=w542, "type"=0.0) -> ("data"=w540:dbl)  [unwired: 1 in, 1 out]
                }
                n237 = local read "Length Array for One week"() -> (w460:dbl[])
                n238 = Array Size(array=w460) -> (size(s)=w457:i32)
                n239 = Greater Than 0?(x=w457) -> (x > 0?=w459:bool)
                n240 = local read "graph refreshed or not"() -> (w456:bool)
                n241 = case shown="False" w459 {
                  tunnel: w458 -> [w521 w523]
                  tunnel: w457 -> [_ w522]
                  frame False {
                    n242 = local write "Length Array for One week"(w521) -> ()
                  }
                  frame True {
                    n243 = for {
                      tunnel: w523 -> [w528] mode=indexing
                      tunnel: w522 -> [w526]
                      i -> [w527]
                      n244 = local read "Length Array for One week"() -> (w529:dbl[])
                      n245 = Add(x=w526, y=w527) -> (x+y=w525:i32)
                      n246 = Insert Into Array(array=w529, index=w525, new element=w528) -> (w524:dbl[])
                      n247 = local write "Length Array for One week"(w524) -> ()
                    }
                  }
                }
                n248 = case shown="True" w456 {
                  frame True {
                    n249 = local write "graph refreshed or not"(FALSE ("graph refreshed or not")) -> ()
                  }
                  frame False {
                    n250 = property on="ZooM" class="XYGraph (strict)"("Value"=cluster{timestamp[], dbl[]} {[], []}) -> ()  [unwired: 2 in, 2 out]
                  }
                }
              }
              frame #1 {
                n251 = local read "DateTime Array for one week"() -> (w624:timestamp[])
                n252 = local read "Length Array for One week"() -> (w625:dbl[])
                n253 = Bundle("DateTime Array for one week"=w624, "Length Array for One week"=w625) -> (w623:T7)  [unwired: 1 in]
                n254 = property on="ZooM" class="XYGraph (strict)"("Value"=w623) -> ()  [unwired: 2 in, 2 out]
              }
            }
          }
        }
      }
      event "One Month": Value Change {
        n255 = event-data() -> ("NewVal"=w630:bool)  [unwired: 1 in, 5 out]
        n256 = And(x=TRUE, y=w630) -> (x .and. y?=w628:bool)
        n257 = case shown="True" w628 {
          tunnel: w627 -> [_ w631]
          tunnel: w626 -> [_ w632]
          frame False {
          }
          frame True {
            n258 = stacked-sequence {
              tunnel: w632 -> [w653 _]
              tunnel: w631 -> [w654 _]
              frame #0 {
                w644 = FALSE ("1Hour")
                n259 = local read "from Date"() -> (w663:timestamp)
                n260 = local read "To Date"() -> (w662:timestamp)
                n261 = local write "1Hour"(w644) -> ()
                n262 = local write "One Day"(w644) -> ()
                n263 = local write "One Week"(w644) -> ()
                n264 = local write "OneMinute"(w644) -> ()
                n265 = local write "30Minute"(w644) -> ()
                n266 = local write "Currently active btn"("one Month ") -> ()
                n267 = Get Date/Time String(seconds (now)=w662) -> (date string=w676:string)  [unwired: 2 in, 1 out]
                n268 = Get Date/Time String(seconds (now)=w663) -> (date string=w657:string)  [unwired: 2 in, 1 out]
                n269 = String Subset(string=w676, offset (0)=6) -> (substring=w675:string)  [unwired: 1 in]
                n270 = String Subset(string=w676, offset (0)=3, length (rest)=2 ("length (rest)")) -> (substring=w673:string)
                n271 = String Subset(string=w676, offset (0)=0, length (rest)=2 ("length (rest)")) -> (substring=w671:string)
                n272 = String Subset(string=w657, offset (0)=6) -> (substring=w655:string)  [unwired: 1 in]
                n273 = String Subset(string=w657, offset (0)=3, length (rest)=2 ("length (rest)")) -> (substring=w659:string)
                n274 = String Subset(string=w657, offset (0)=0, length (rest)=2 ("length (rest)")) -> (substring=w665:string)
                n275 = Concatenate Strings(w675, "-" ("string"), w673, "-" ("string"), w671) -> (w670:string)
                n276 = Concatenate Strings(w655, "-" ("string"), w659, "-" ("string"), w665) -> (w664:string)
                n277 = Concatenate Strings("SELECT \n        DATEADD(month, (DATEDIFF(month , " ("string"), " ' " ("string"), w664, "  ' , " ("string"), "DateTime) ) , " ("string"), "'  " ("string"), w664, " ')  " ("string"), " AS  Per_Month_interval,\n        AVG(Length) AS avg_length\n    FROM \n        DataAnaysis\n    WHERE \n        DateTime >=  '" ("string"), w664, "' AND DateTime <  '  " ("string"), w670, "  ' " ("string"), " GROUP BY  " ("string"), "DATEADD(month, (DATEDIFF(month, ' " ("string"), w664, " ' " ("string"), " , DateTime) ) ,  ' " ("string"), w664, "  ' )" ("string"), "ORDER BY \n        Per_Month_interval; " ("string")) -> (w650:string)
                "concatenated string 8" <- w650
                n278 = call-poly <vilib>:"DB Tools Execute Query.vi"("error in (no error)"=w654, "SQL query"=w650, "connection reference"=w653) -> ("error out"=w652:errorcluster, "recordset reference"=w651:T5)  [unwired: 5 in]
                n279 = local read "DateTime Array for One Month"() -> (w643:timestamp[])
                n280 = call-poly <vilib>:"DB Tools Fetch Recordset Data.vi"("error in (no error)"=w652, "recordset reference"=w651) -> ("recordset data"=w645:variant[][])  [unwired: 3 in, 2 out]
                n281 = Index Array(array=w645, index (col)=1 ("disabled index (col)")) -> (element=w646:variant[])  [unwired: 1 in]
                n282 = Index Array(array=w645, index (col)=0 ("disabled index (col)")) -> (element=w648:variant[])  [unwired: 1 in]
                n283 = Array Size(array=w643) -> (size(s)=w639:i32)
                n284 = Greater Than 0?(x=w639) -> (x > 0?=w642:bool)
                n285 = local read "graph refreshed or not"() -> (w633:bool)
                n286 = for {
                  tunnel: w648 -> [w755] mode=indexing
                  tunnel: [w753] -> w640 mode=indexing
                  n287 = xnode "Database Variant To Data"("database variant"=w755, "type"=timestamp(0 s since 1904-01-01)) -> ("data"=w753:timestamp)  [unwired: 1 in, 1 out]
                }
                n288 = case shown="True" w633 {
                  frame False {
                    n289 = property on="ZooM" class="XYGraph (strict)"("Value"=cluster{timestamp[], dbl[]} {[], []}) -> ()  [unwired: 2 in, 2 out]
                  }
                  frame True {
                    n290 = local write "graph refreshed or not"(FALSE ("graph refreshed or not")) -> ()
                  }
                }
                n291 = Array Size(array=w640) -> (size(s)=w641:i32)
                n292 = case shown="True" w642 {
                  tunnel: w641 -> [_ w711]
                  tunnel: w640 -> [w708 w710]
                  tunnel: w639 -> [_ w709]
                  frame False {
                    n293 = local write "DateTime Array for One Month"(w708) -> ()
                  }
                  frame True {
                    n294 = for {
                      N: w711 -> [_]
                      tunnel: w710 -> [w717] mode=indexing
                      tunnel: w709 -> [w714]
                      i -> [w715]
                      n295 = local read "DateTime Array for One Month"() -> (w716:timestamp[])
                      n296 = Add(x=w714, y=w715) -> (x+y=w713:i32)
                      n297 = Insert Into Array(array=w716, index=w713, new element=w717) -> (w712:timestamp[])
                      n298 = local write "DateTime Array for One Month"(w712) -> ()
                    }
                  }
                }
                n299 = local read "Length Array for One Month"() -> (w638:dbl[])
                n300 = Array Size(array=w638) -> (size(s)=w635:i32)
                n301 = Greater Than 0?(x=w635) -> (x > 0?=w637:bool)
                n302 = for {
                  tunnel: w646 -> [w720] mode=indexing
                  tunnel: [w718] -> w634 mode=indexing
                  n303 = xnode "Database Variant To Data"("database variant"=w720, "type"=0.0) -> ("data"=w718:dbl)  [unwired: 1 in, 1 out]
                }
                n304 = Array Size(array=w634) -> (size(s)=w636:i32)
                n305 = case shown="True" w637 {
                  tunnel: w636 -> [_ w701]
                  tunnel: w635 -> [_ w700]
                  tunnel: w634 -> [_ w699]
                  frame False {
                  }
                  frame True {
                    n306 = for {
                      N: w701 -> [_]
                      tunnel: w700 -> [w706]
                      tunnel: w699 -> [w704] mode=indexing
                      i -> [w707]
                      n307 = local read "Length Array for One Month"() -> (w703:dbl[])
                      n308 = Add(x=w706, y=w707) -> (x+y=w705:i32)
                      n309 = Insert Into Array(array=w703, index=w705, new element=w704) -> (w702:dbl[])
                      n310 = local write "Length Array for One Month"(w702) -> ()
                    }
                  }
                }
              }
              frame #1 {
                n311 = local read "DateTime Array for One Month"() -> (w802:timestamp[])
                n312 = local read "Length Array for One Month"() -> (w803:dbl[])
                n313 = Bundle("DateTime Array for One Month"=w802, "Length Array for One Month"=w803) -> (w801:T8)  [unwired: 1 in]
                n314 = property on="ZooM" class="XYGraph (strict)"("Value"=w801) -> ()  [unwired: 2 in, 2 out]
              }
            }
          }
        }
      }
      event "1Hour": Value Change {
        n315 = event-data() -> ("NewVal"=w808:bool)  [unwired: 1 in, 5 out]
        n316 = And(x=TRUE, y=w808) -> (x .and. y?=w806:bool)
        n317 = case shown="True" w806 {
          tunnel: w805 -> [_ w809]
          tunnel: w804 -> [_ w810]
          frame False {
          }
          frame True {
            n318 = stacked-sequence {
              tunnel: w810 -> [w831 _]
              tunnel: w809 -> [w832 _]
              frame #0 {
                w822 = FALSE ("30Minute")
                n319 = local read "from Date"() -> (w835:timestamp)
                n320 = local read "To Date"() -> (w834:timestamp)
                n321 = local write "30Minute"(w822) -> ()
                n322 = local write "One Day"(w822) -> ()
                n323 = local write "One Month"(w822) -> ()
                n324 = local write "One Week"(w822) -> ()
                n325 = local write "OneMinute"(w822) -> ()
                n326 = local write "Currently active btn"("1Hour ") -> ()
                n327 = Get Date/Time String(seconds (now)=w834) -> (date string=w854:string)  [unwired: 2 in, 1 out]
                n328 = Get Date/Time String(seconds (now)=w835) -> (date string=w837:string)  [unwired: 2 in, 1 out]
                n329 = String Subset(string=w854, offset (0)=6) -> (substring=w853:string)  [unwired: 1 in]
                n330 = String Subset(string=w854, offset (0)=3, length (rest)=2 ("length (rest)")) -> (substring=w851:string)
                n331 = String Subset(string=w854, offset (0)=0, length (rest)=2 ("length (rest)")) -> (substring=w849:string)
                n332 = String Subset(string=w837, offset (0)=6) -> (substring=w842:string)  [unwired: 1 in]
                n333 = String Subset(string=w837, offset (0)=3, length (rest)=2 ("length (rest)")) -> (substring=w840:string)
                n334 = String Subset(string=w837, offset (0)=0, length (rest)=2 ("length (rest)")) -> (substring=w838:string)
                n335 = Concatenate Strings(w853, "-" ("string"), w851, "-" ("string"), w849) -> (w848:string)
                n336 = Concatenate Strings(w842, "-" ("string"), w840, "-" ("string"), w838) -> (w836:string)
                n337 = Concatenate Strings("SELECT \n        DATEADD(hour, (DATEDIFF(hour, " ("string"), " ' " ("string"), w836, "  ' , " ("string"), "DateTime) ) , " ("string"), "'  " ("string"), w836, " ')  " ("string"), " AS  Per_hour_interval,\n        AVG(Length) AS avg_length\n    FROM \n        DataAnaysis\n    WHERE \n        DateTime >=  '" ("string"), w836, "' AND DateTime <  '  " ("string"), w848, "  ' " ("string"), " GROUP BY  " ("string"), "DATEADD(hour, (DATEDIFF(hour, ' " ("string"), w836, " ' " ("string"), " , DateTime) ) ,  ' " ("string"), w836, "  ' )" ("string"), "ORDER BY \n        Per_hour_interval; " ("string")) -> (w830:string)
                "concatenated string 5" <- w830
                n338 = call-poly <vilib>:"DB Tools Execute Query.vi"("error in (no error)"=w832, "SQL query"=w830, "connection reference"=w831) -> ("error out"=w829:errorcluster, "recordset reference"=w828:T5)  [unwired: 5 in]
                n339 = call-poly <vilib>:"DB Tools Fetch Recordset Data.vi"("error in (no error)"=w829, "recordset reference"=w828) -> ("recordset data"=w825:variant[][])  [unwired: 3 in, 2 out]
                n340 = Index Array(array=w825, index (col)=1 ("disabled index (col)")) -> (element=w826:variant[])  [unwired: 1 in]
                n341 = Index Array(array=w825, index (col)=0 ("disabled index (col)")) -> (element=w823:variant[])  [unwired: 1 in]
                n342 = for {
                  tunnel: w823 -> [w899] mode=indexing
                  tunnel: [w897] -> w812 mode=indexing
                  n343 = xnode "Database Variant To Data"("database variant"=w899, "type"=timestamp(0 s since 1904-01-01)) -> ("data"=w897:timestamp)  [unwired: 1 in, 1 out]
                }
                n344 = local read "graph refreshed or not"() -> (w811:bool)
                n345 = for {
                  tunnel: w826 -> [w947] mode=indexing
                  tunnel: [w945] -> w817 mode=indexing
                  n346 = xnode "Database Variant To Data"("database variant"=w947, "type"=0.0) -> ("data"=w945:dbl)  [unwired: 1 in, 1 out]
                }
                n347 = local read "DateTime Array for 1 Hour"() -> (w816:timestamp[])
                n348 = local read "Length Array for 1 Hour"() -> (w821:dbl[])
                n349 = case shown="True" w811 {
                  frame True {
                    n350 = local write "graph refreshed or not"(FALSE ("graph refreshed or not")) -> ()
                  }
                  frame False {
                    n351 = property on="ZooM" class="XYGraph (strict)"("Value"=cluster{timestamp[], dbl[]} {[], []}) -> ()  [unwired: 2 in, 2 out]
                  }
                }
                n352 = Array Size(array=w812) -> (size(s)=w814:i32)
                n353 = Array Size(array=w817) -> (size(s)=w819:i32)
                n354 = Array Size(array=w816) -> (size(s)=w813:i32)
                n355 = Greater Than 0?(x=w813) -> (x > 0?=w815:bool)
                n356 = Array Size(array=w821) -> (size(s)=w818:i32)
                n357 = Greater Than 0?(x=w818) -> (x > 0?=w820:bool)
                n358 = case shown="True" w815 {
                  tunnel: w814 -> [_ w880]
                  tunnel: w813 -> [_ w879]
                  tunnel: w812 -> [w877 w878]
                  frame False {
                    n359 = local write "DateTime Array for 1 Hour"(w877) -> ()
                  }
                  frame True {
                    n360 = for {
                      N: w880 -> [_]
                      tunnel: w879 -> [w885]
                      tunnel: w878 -> [w883] mode=indexing
                      i -> [w886]
                      n361 = local read "DateTime Array for 1 Hour"() -> (w882:timestamp[])
                      n362 = Add(x=w885, y=w886) -> (x+y=w884:i32)
                      n363 = Insert Into Array(array=w882, index=w884, new element=w883) -> (w881:timestamp[])
                      n364 = local write "DateTime Array for 1 Hour"(w881) -> ()
                    }
                  }
                }
                n365 = case shown="True" w820 {
                  tunnel: w819 -> [_ w890]
                  tunnel: w818 -> [_ w889]
                  tunnel: w817 -> [w887 w888]
                  frame False {
                    n366 = local write "Length Array for 1 Hour"(w887) -> ()
                  }
                  frame True {
                    n367 = for {
                      N: w890 -> [_]
                      tunnel: w889 -> [w894]
                      tunnel: w888 -> [w892] mode=indexing
                      i -> [w895]
                      n368 = Add(x=w894, y=w895) -> (x+y=w893:i32)
                      n369 = local read "Length Array for 1 Hour"() -> (w896:dbl[])
                      n370 = Insert Into Array(array=w896, index=w893, new element=w892) -> (w891:dbl[])
                      n371 = local write "Length Array for 1 Hour"(w891) -> ()
                    }
                  }
                }
              }
              frame #1 {
                n372 = local read "DateTime Array for 1 Hour"() -> (w981:timestamp[])
                n373 = local read "Length Array for 1 Hour"() -> (w982:dbl[])
                n374 = Bundle("DateTime Array for 1 Hour"=w981, "Length Array for 1 Hour"=w982) -> (w980:T9)  [unwired: 1 in]
                n375 = property on="ZooM" class="XYGraph (strict)"("Value"=w980) -> ()  [unwired: 2 in, 2 out]
              }
            }
          }
        }
      }
      event "One Day": Value Change {
        n376 = event-data() -> ("NewVal"=w987:bool)  [unwired: 1 in, 5 out]
        n377 = And(x=TRUE, y=w987) -> (x .and. y?=w985:bool)
        n378 = case shown="True" w985 {
          tunnel: w984 -> [_ w988]
          tunnel: w983 -> [_ w989]
          frame False {
          }
          frame True {
            n379 = stacked-sequence {
              tunnel: w989 -> [w1008 _]
              tunnel: w988 -> [w1009 _]
              frame #0 {
                w999 = FALSE ("1Hour")
                n380 = local read "from Date"() -> (w1013:timestamp)
                n381 = local read "To Date"() -> (w1012:timestamp)
                n382 = local write "1Hour"(w999) -> ()
                n383 = local write "Currently active btn"("One Day ") -> ()
                n384 = local read "graph refreshed or not"() -> (w990:bool)
                n385 = local write "One Month"(w999) -> ()
                n386 = local write "One Week"(w999) -> ()
                n387 = local write "OneMinute"(w999) -> ()
                n388 = local write "30Minute"(w999) -> ()
                n389 = Get Date/Time String(seconds (now)=w1012) -> (date string=w1031:string)  [unwired: 2 in, 1 out]
                n390 = Get Date/Time String(seconds (now)=w1013) -> (date string=w1010:string)  [unwired: 2 in, 1 out]
                n391 = String Subset(string=w1031, offset (0)=6) -> (substring=w1030:string)  [unwired: 1 in]
                n392 = String Subset(string=w1031, offset (0)=3, length (rest)=2 ("length (rest)")) -> (substring=w1028:string)
                n393 = String Subset(string=w1031, offset (0)=0, length (rest)=2 ("length (rest)")) -> (substring=w1026:string)
                n394 = String Subset(string=w1010, offset (0)=6) -> (substring=w1019:string)  [unwired: 1 in]
                n395 = String Subset(string=w1010, offset (0)=3, length (rest)=2 ("length (rest)")) -> (substring=w1017:string)
                n396 = String Subset(string=w1010, offset (0)=0, length (rest)=2 ("length (rest)")) -> (substring=w1015:string)
                n397 = case shown="True" w990 {
                  frame True {
                    n398 = local write "graph refreshed or not"(FALSE ("graph refreshed or not")) -> ()
                  }
                  frame False {
                    n399 = local write "graph refreshed or not"(FALSE ("graph refreshed or not")) -> ()
                    n400 = property on="ZooM" class="XYGraph (strict)"("Value"=cluster{timestamp[], dbl[]} {[], []}) -> ()  [unwired: 2 in, 2 out]
                  }
                }
                n401 = Concatenate Strings(w1030, "-" ("string"), w1028, "-" ("string"), w1026) -> (w1025:string)
                n402 = Concatenate Strings(w1019, "-" ("string"), w1017, "-" ("string"), w1015) -> (w1014:string)
                n403 = Concatenate Strings("SELECT \n        DATEADD(day, (DATEDIFF(day , " ("string"), " ' " ("string"), w1014, "  ' , " ("string"), "DateTime) ) , " ("string"), "'  " ("string"), w1014, " ')  " ("string"), " AS  Per_day_interval,\n        AVG(Length) AS avg_length\n    FROM \n        DataAnaysis\n    WHERE \n        DateTime >=  '" ("string"), w1014, "' AND DateTime <  '  " ("string"), w1025, "  ' " ("string"), " GROUP BY  " ("string"), "DATEADD(day, (DATEDIFF(day, ' " ("string"), w1014, " ' " ("string"), " , DateTime) ) ,  ' " ("string"), w1014, "  ' )" ("string"), "ORDER BY \n        Per_day_interval; " ("string")) -> (w1007:string)
                "concatenated string 6" <- w1007
                n404 = call-poly <vilib>:"DB Tools Execute Query.vi"("error in (no error)"=w1009, "SQL query"=w1007, "connection reference"=w1008) -> ("error out"=w1005:errorcluster, "recordset reference"=w1006:T5)  [unwired: 5 in]
                n405 = call-poly <vilib>:"DB Tools Fetch Recordset Data.vi"("error in (no error)"=w1005, "recordset reference"=w1006) -> ("recordset data"=w1000:variant[][])  [unwired: 3 in, 2 out]
                n406 = local read "Length Array for 1 Day"() -> (w992:dbl[])
                n407 = Index Array(array=w1000, index (col)=1 ("disabled index (col)")) -> (element=w1003:variant[])  [unwired: 1 in]
                n408 = Index Array(array=w1000, index (col)=0 ("disabled index (col)")) -> (element=w1001:variant[])  [unwired: 1 in]
                n409 = local read "DateTime Array for 1 Day"() -> (w991:timestamp[])
                n410 = for {
                  tunnel: w1003 -> [w1125] mode=indexing
                  tunnel: [w1123] -> w997 mode=indexing
                  n411 = xnode "Database Variant To Data"("database variant"=w1125, "type"=0.0) -> ("data"=w1123:dbl)  [unwired: 1 in, 1 out]
                }
                n412 = for {
                  tunnel: w1001 -> [w1077] mode=indexing
                  tunnel: [w1075] -> w994 mode=indexing
                  n413 = xnode "Database Variant To Data"("database variant"=w1077, "type"=timestamp(0 s since 1904-01-01)) -> ("data"=w1075:timestamp)  [unwired: 1 in, 1 out]
                }
                n414 = Array Size(array=w992) -> (size(s)=w996:i32)
                n415 = Greater Than 0?(x=w996) -> (x > 0?=w998:bool)
                n416 = case shown="True" w998 {
                  tunnel: w997 -> [w1065 w1067]
                  tunnel: w996 -> [_ w1068]
                  frame False {
                    n417 = local write "Length Array for 1 Day"(w1065) -> ()
                  }
                  frame True {
                    n418 = Array Size(array=w1067) -> (size(s)=w1066:i32)
                    n419 = for {
                      N: w1066 -> [_]
                      tunnel: w1067 -> [w1074] mode=indexing
                      tunnel: w1068 -> [w1072]
                      i -> [w1073]
                      n420 = Add(x=w1073, y=w1072) -> (x+y=w1071:i32)
                      n421 = local read "Length Array for 1 Day"() -> (w1070:dbl[])
                      n422 = Insert Into Array(array=w1070, index=w1071, new element=w1074) -> (w1069:dbl[])
                      n423 = local write "Length Array for 1 Day"(w1069) -> ()
                    }
                  }
                }
                n424 = Array Size(array=w991) -> (size(s)=w993:i32)
                n425 = Greater Than 0?(x=w993) -> (x > 0?=w995:bool)
                n426 = case shown="True" w995 {
                  tunnel: w991 -> [_ _]
                  tunnel: w994 -> [w1055 w1056]
                  tunnel: w993 -> [_ w1058]
                  frame False {
                    n427 = local write "DateTime Array for 1 Day"(w1055) -> ()
                  }
                  frame True {
                    n428 = Array Size(array=w1056) -> (size(s)=w1057:i32)
                    n429 = for {
                      N: w1057 -> [_]
                      tunnel: w1056 -> [w1061] mode=indexing
                      tunnel: w1058 -> [w1063]
                      i -> [w1064]
                      n430 = Add(x=w1064, y=w1063) -> (x+y=w1060:i32)
                      n431 = local read "DateTime Array for 1 Day"() -> (w1062:timestamp[])
                      n432 = Insert Into Array(array=w1062, index=w1060, new element=w1061) -> (w1059:timestamp[])
                      n433 = local write "DateTime Array for 1 Day"(w1059) -> ()
                    }
                  }
                }
              }
              frame #1 {
                n434 = local read "DateTime Array for 1 Day"() -> (w1159:timestamp[])
                n435 = local read "Length Array for 1 Day"() -> (w1160:dbl[])
                n436 = Bundle("DateTime Array for 1 Day"=w1159, "Length Array for 1 Day"=w1160) -> (w1158:T10)  [unwired: 1 in]
                n437 = property on="ZooM" class="XYGraph (strict)"("Value"=w1158) -> ()  [unwired: 2 in, 2 out]
              }
            }
          }
        }
      }
    }
    n438 = local read "Stop Button"() -> (w76:bool)
    n439 = And(x=TRUE, y=w76) -> (x .and. y?=w75:bool)
  }
  n440 = stacked-sequence {
    frame #0 {
    }
    frame #1 {
      w1161 = FALSE ("graph refreshed or not")
      w1163 = dbl[] [] ("Length Array")
      w1162 = timestamp[] [] ("DateTime Array for 1 Day")
      w1164 = FALSE ("One Day")
      n441 = local write "Currently active btn"(" " ("Currently active btn")) -> ()
      n442 = local write "OneMinute"(w1164) -> ()
      n443 = local write "One Week"(w1164) -> ()
      n444 = local write "One Month"(w1164) -> ()
      n445 = local write "30Minute"(w1164) -> ()
      n446 = local write "DateTime Array for 1 Hour"(w1162) -> ()
      n447 = local write "DateTime Array for One Month"(w1162) -> ()
      n448 = local write "DateTime Array for one week"(w1162) -> ()
      n449 = local write "1Hour"(w1164) -> ()
      n450 = local write "DateTime Array for 30 mins"(w1162) -> ()
      n451 = local write "One Day"(w1164) -> ()
      n452 = local write "DateTime Array for 1 Day"(w1162) -> ()
      n453 = local write "DateTime Array"(w1162) -> ()
      n454 = local write "graph refreshed or not"(w1161) -> ()
      n455 = local write "Length Array for 1 Day"(w1163) -> ()
      n456 = local write "Length Array for 30 mins"(w1163) -> ()
      n457 = local write "Length Array for One Month"(w1163) -> ()
      n458 = local write "Length Array for One week"(w1163) -> ()
      n459 = local write "Length Array for 1 Hour"(w1163) -> ()
      n460 = local write "Stop Button"(w1161) -> ()
      n461 = local write "Length Array"(w1163) -> ()
    }
  }
